vi "System Log Consumer Loop.vi"(0 "Stop Program":refnum<vi>, 1 "System Queue":refnum<vi>, 2 "System Visual Log":refnum<vi>) -> ()   [LabVIEW 2022 SP3]
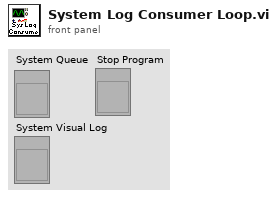
[diagram p1: front panel]
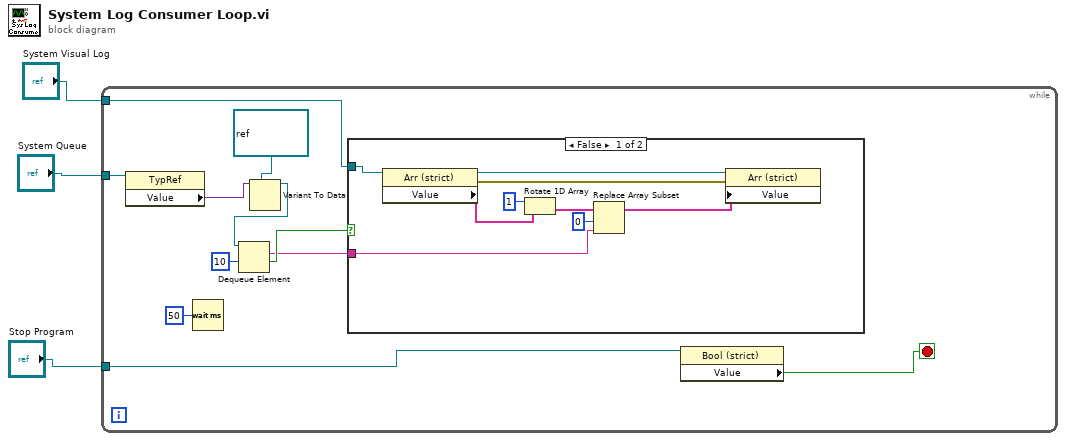
[diagram p0: block diagram]
diagram:
  n1 = while {
    tunnel: "System Queue" -> [w10]
    tunnel: "System Visual Log" -> [w8]
    tunnel: "Stop Program" -> [w7]
    stop <- w5 stop-if-true
    n2 = property class="TypRef"(reference=w10) -> ("Value"=w12:variant)  [unwired: 1 in, 2 out]
    n3 = Wait (ms)(milliseconds to wait=u32 50) -> ()  [unwired: 1 out]
    n4 = Variant To Data(type=refnum<queue> refnum ("Queue Reactor 6"), Variant=w12) -> (data=w9:refnum<queue>)  [unwired: 1 in, 1 out]
    n5 = Dequeue Element(queue=w9, timeout in ms (-1)=10) -> (element=w13:string, timed out?=w14:bool)  [unwired: 1 in, 2 out]
    n6 = case shown="False" w14 {
      tunnel: w13 -> [w20 _]
      tunnel: w8 -> [w17 _]
      frame False {
        n7 = property class="Arr (strict)"(reference=w17) -> (reference out=w16:refnum<vi>, error out=w15:errorcluster, "Value"=w19:string[])  [unwired: 1 in]
        n8 = Rotate 1D Array(1:w19, 2:1 ("n")) -> (0:w22:string[])
        n9 = Replace Array Subset(array=w22, new element=w20, index=0) -> (w18:string[])
        n10 = property class="Arr (strict)"(reference=w16, error in=w15, "Value"=w18) -> ()  [unwired: 2 out]
      }
      frame True {
        # "Nothing present. Wait for next log."
      }
    }
    n11 = property class="Bool (strict)"(reference=w7) -> ("Value"=w5:bool)  [unwired: 1 in, 2 out]
  }
